vi "Stand-Alone Detect High Current - Prevent Trip.vi"() -> ()   [LabVIEW 2020]
panel:
  in  "stop":bool
  out "Mesurnment Iteration":i32
  out "Actual Current Limit (nA)":dbl format="%#_13g"
  out "Power Supply Trip":bool
  out "Actual Voltage Level (V)":dbl format="%#_13g"
  in  "Power Supply \nAddress":refnum<visa-resource-name>
  in  "Barcodes in":string[](array[string])
  in  "Barcodes in 2":string[](array[string])
  in  "Barcodes in 3":string[](array[string])
  in  "Barcodes in 4":string[](array[string])
  out "Elapsed Time (s)":dbl
  in  "Start":bool
  out "Test Is Running (Red)\nTest Is Stopped (Green)":bool
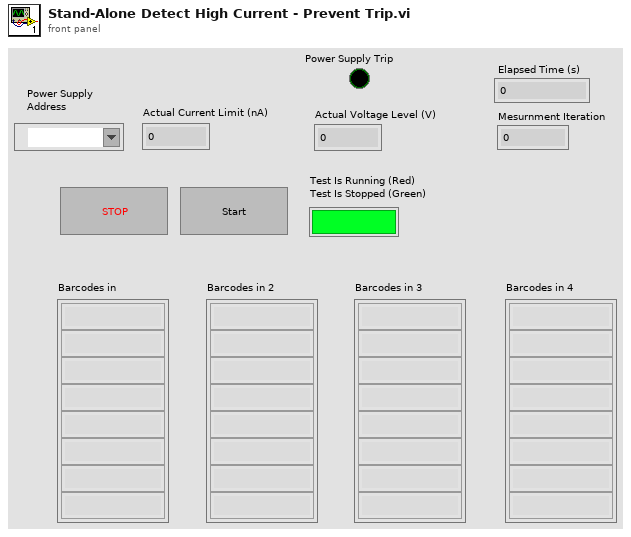
[diagram p1: front panel]
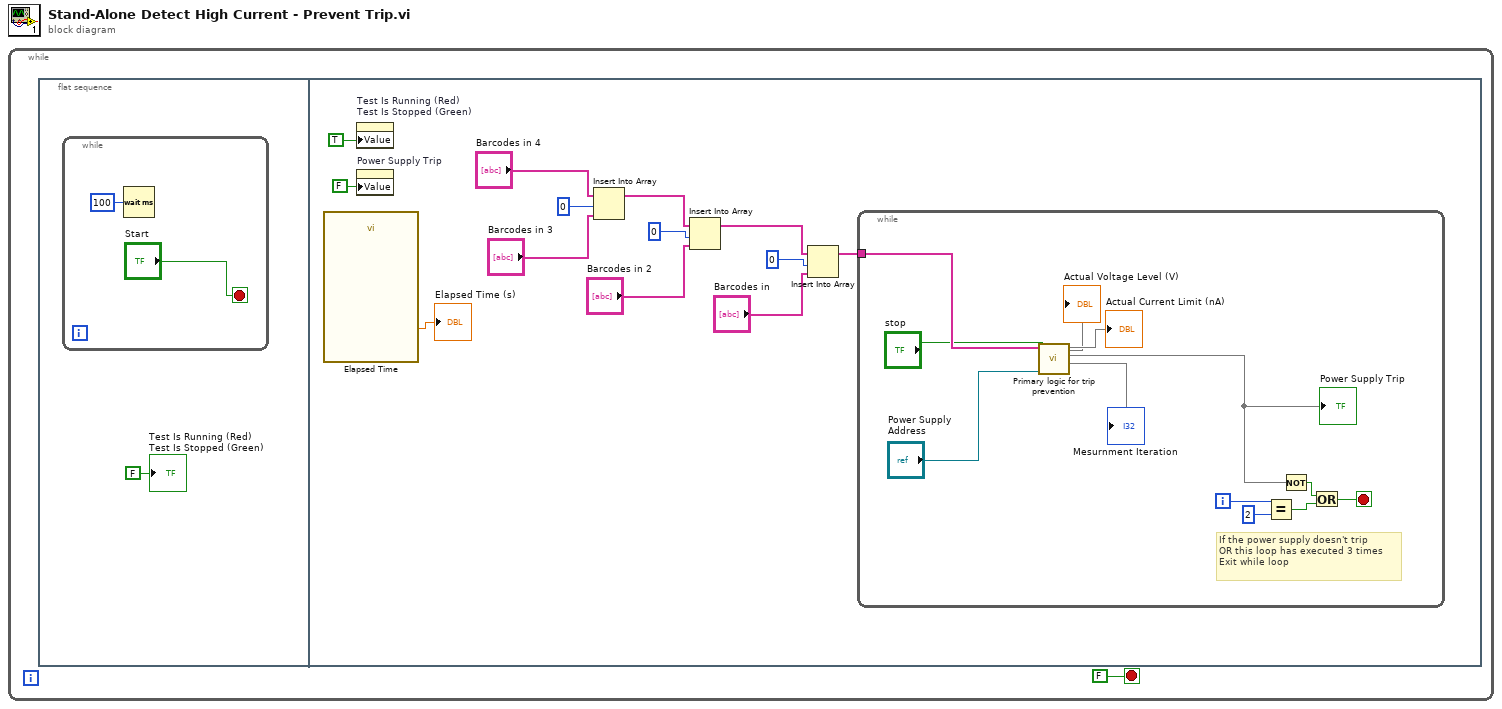
[diagram p0: block diagram]
diagram:
  n1 = while {
    stop <- FALSE stop-if-true
    n2 = flat-sequence {
      frame #0 {
        n3 = while {
          stop <- "Start" stop-if-true
          n4 = Wait (ms)(milliseconds to wait=u32 100) -> ()  [unwired: 1 out]
        }
        "Test Is Running (Red)\nTest Is Stopped (Green)" <- FALSE ("Start LED")
      }
      frame #1 {
        n5 = call "Elapsed Time"() -> ("Elapsed Time (s)"=→"Elapsed Time (s)":dbl)  [unwired: 12 in, 7 out]
        n6 = property on="Test Is Running (Red)\nTest Is Stopped (Green)" class="Bool (strict)"("Value"=TRUE) -> ()  [unwired: 2 in, 2 out]
        n7 = property on="Power Supply Trip" class="Bool (strict)"("Value"=FALSE ("Power Supply Trip")) -> ()  [unwired: 2 in, 2 out]
        n8 = Insert Into Array(array="Barcodes in 4", index=0, new element="Barcodes in 3") -> (w11:string[])
        n9 = Insert Into Array(array=w11, index=0, new element="Barcodes in 2") -> (w7:string[])
        n10 = Insert Into Array(array=w7, index=0, new element="Barcodes in") -> (w6:string[])
        n11 = while {
          tunnel: w6 -> [w24]
          i -> [w28]
          stop <- w25 stop-if-true
          # "If the power supply doesn't trip\nOR this loop has executed 3 times Exit while loop"
          n12 = call "Primary logic for trip prevention.vi"("VISA Refnum in"="Power Supply \nAddress", 10:"stop", 11:w24) -> (2:w20, 3:→"Actual Current Limit (nA)", 4:→"Mesurnment Iteration", 5:→"Actual Voltage Level (V)")  [unwired: 5 in]
          "Power Supply Trip" <- w20
          n13 = Equal?(x=w28, y=2) -> (x = y?=w26:bool)
          n14 = Not(x=w20) -> (.not. x?=w29:bool)
          n15 = Or(x=w29, y=w26) -> (x .or. y?=w25:bool)
        }
      }
    }
  }
